vi "Calculate View Matrix.vi"(10 "Camera Rotation":sgl, 11 "Camera Position":T1) -> (3 "View Matrix":sgl[][](array[numeric]))   [LabVIEW 2020, in "3D.lvlib"]
uses:
  3D.lvlib
  Vector 3D.ctl
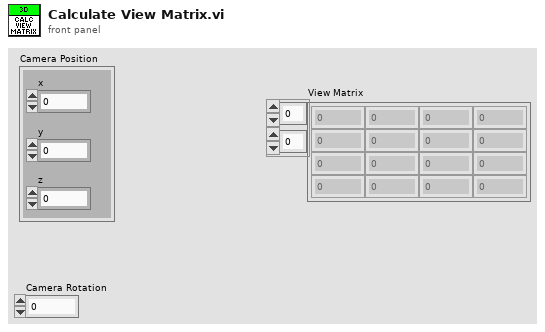
[diagram p1: front panel]
types:
  T1 = typedef "3D.lvlib/Vector 3D.ctl" = cluster{"x":sgl, "y":sgl, "z":sgl}
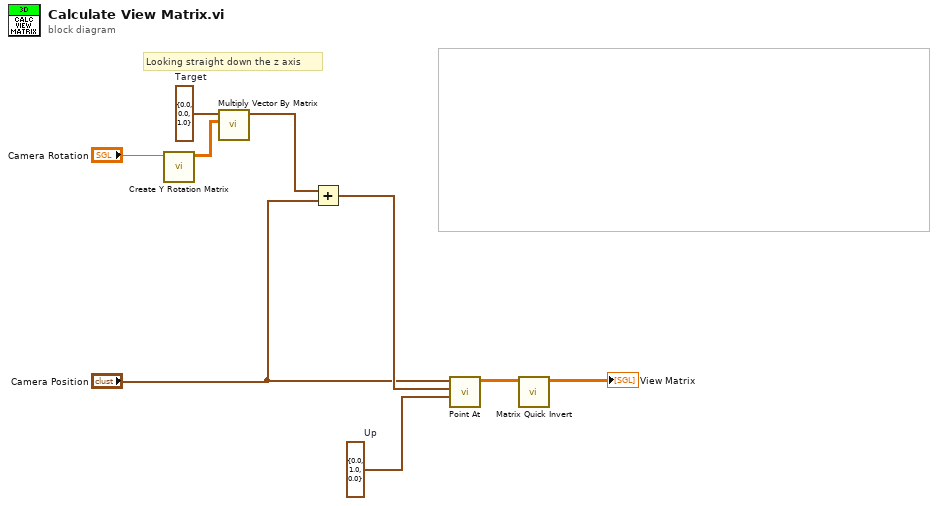
[diagram p0: block diagram]
diagram:
  w5 = T1 {"x"=0.0, "y"=1.0, "z"=0.0}  # Up
  w9 = T1 {"x"=0.0, "y"=0.0, "z"=1.0}  # Target
  # "Looking straight down the z axis"
  n1 = call "Create Y Rotation Matrix.vi"("Theta (°)"="Camera Rotation") -> ("Rotation Y Matrix"=w8:sgl[][])  [unwired: 10 in]
  n2 = call "Multiply Vector By Matrix.vi"("Matrix in"=w8, "Vector 3D in"=w9) -> ("Vector 3D out"=w7:T1)  [unwired: 9 in]
  n3 = Add(x=w7, y="Camera Position") -> (x+y=w6:T1)
  n4 = call "Point At.vi"("Up"=w5, "Target"=w6, "Position"="Camera Position") -> ("Point At Matrix"=w4:sgl[][])  [unwired: 8 in]
  n5 = call "Matrix Quick Invert.vi"("Matrix"=w4) -> ("Matrix Inverted"=→"View Matrix":sgl[][])  [unwired: 10 in]
